vi "读取临时表格数据 (子VI).vi"(8 "time 2":string, 9 "表格选择":string(combo)="database1.mdb", 10 "组合框":string(combo), 11 "String输入":refnum<vi>) -> ()   [LabVIEW 2016]
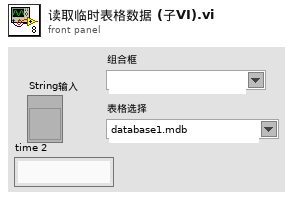
[diagram p1: front panel]
types:
  T1 = enum16{"CODMn", "PH", "氨氮", "总氮", "总磷", "CODCr", "电导率", "水温", "DO", "浊度", "叶绿素", "藻密度"}
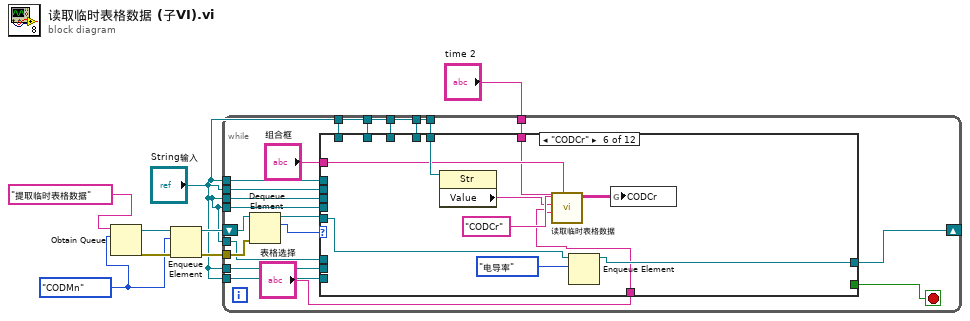
[diagram p0: block diagram]
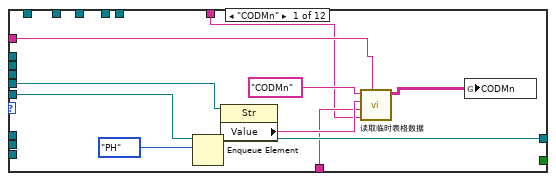
[diagram p2: hidden frame]
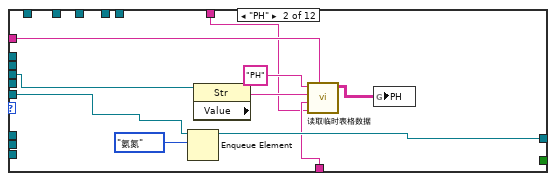
[diagram p3: hidden frame]
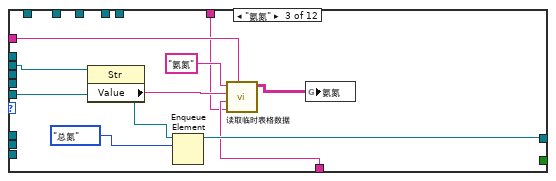
[diagram p4: hidden frame]
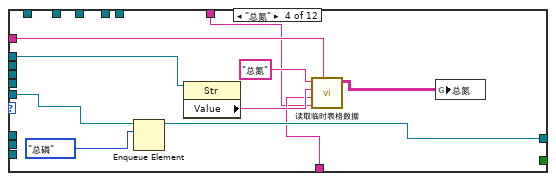
[diagram p5: hidden frame]
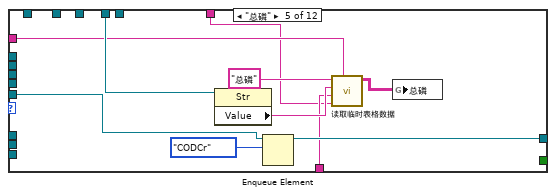
[diagram p6: hidden frame]
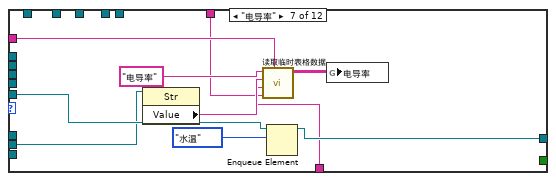
[diagram p7: hidden frame]
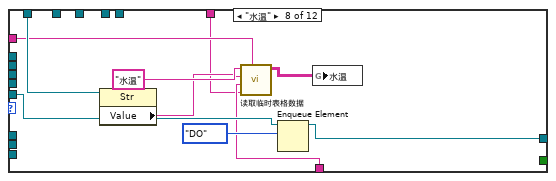
[diagram p8: hidden frame]
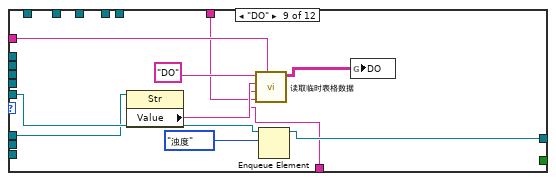
[diagram p9: hidden frame]
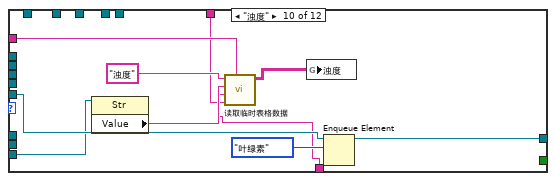
[diagram p10: hidden frame]
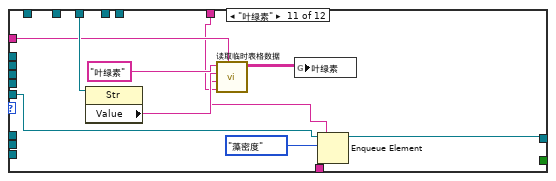
[diagram p11: hidden frame]
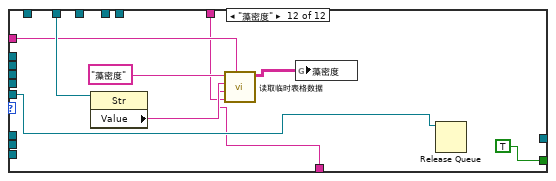
[diagram p12: hidden frame]
diagram:
  w4 = T1."CODMn"
  n1 = Obtain Queue(name (unnamed)="提取临时表格数据" ("新元素/子数组"), element data type=w4) -> (queue out=w8:refnum<queue>, error out=w5:errorcluster)  [unwired: 3 in, 1 out]
  n2 = Enqueue Element(queue=w8, element=w4, error in (no error)=w5) -> (queue out=w7:refnum<queue>, error out=w6:errorcluster)  [unwired: 1 in, 1 out]
  n3 = while {
    shift-right: [w27] -> _
    shift-left: w7 -> [w29]
    tunnel: w6 -> [w26]
    tunnel: "String输入" -> [w23]
    tunnel: "String输入" -> [w22]
    tunnel: "String输入" -> [w21]
    tunnel: "String输入" -> [w20]
    tunnel: "String输入" -> [w19]
    tunnel: "String输入" -> [w18]
    tunnel: "String输入" -> [w17]
    tunnel: "String输入" -> [w16]
    tunnel: "String输入" -> [w15]
    tunnel: "String输入" -> [w14]
    tunnel: "String输入" -> [w13]
    tunnel: "String输入" -> [w12]
    tunnel: "time 2" -> [w9]
    stop <- w24 stop-if-true
    n4 = Dequeue Element(queue=w29, error in (no error)=w26) -> (queue out=w28:refnum<queue>, element=w25:T1)  [unwired: 1 in, 2 out]
    n5 = case shown="\"CODCr\"" w25 {
      tunnel: w28 -> [w39 w49 w58 w69 w78 w88 w98 w108 w118 w128 w138 w147]
      tunnel: [w38 w48 w59 w68 w77 w87 w97 w107 w117 w127 w137 _] -> w27
      tunnel: [_ _ _ _ _ _ _ _ _ _ _ TRUE] -> w24
      tunnel: w23 -> [w33 _ _ _ _ _ _ _ _ _ _ _]
      tunnel: w22 -> [_ w43 _ _ _ _ _ _ _ _ _ _]
      tunnel: w21 -> [_ _ w53 _ _ _ _ _ _ _ _ _]
      tunnel: w20 -> [_ _ _ w63 _ _ _ _ _ _ _ _]
      tunnel: w19 -> [_ _ _ _ w73 _ _ _ _ _ _ _]
      tunnel: w18 -> [_ _ _ _ _ w83 _ _ _ _ _ _]
      tunnel: w17 -> [_ _ _ _ _ _ w93 _ _ _ _ _]
      tunnel: w16 -> [_ _ _ _ _ _ _ w103 _ _ _ _]
      tunnel: w15 -> [_ _ _ _ _ _ _ _ w113 _ _ _]
      tunnel: w14 -> [_ _ _ _ _ _ _ _ _ w123 _ _]
      tunnel: w13 -> [_ _ _ _ _ _ _ _ _ _ w133 _]
      tunnel: w12 -> [_ _ _ _ _ _ _ _ _ _ _ w143]
      tunnel: "组合框" -> [w32 w42 w52 w62 w72 w82 w92 w102 w112 w122 w132 w142]
      tunnel: "表格选择" -> [w31 w41 w51 w61 w71 w81 w91 w101 w111 w121 w131 w141]
      tunnel: w9 -> [w30 w40 w50 w60 w70 w80 w90 w100 w110 w120 w130 w140]
      frame "CODMn" {
        n6 = Enqueue Element(queue=w39, element=T1."PH") -> (queue out=w38:refnum<queue>)  [unwired: 2 in, 2 out]
        n7 = property class="Str"(reference=w33) -> ("Value"=w35:string)  [unwired: 1 in, 2 out]
        n8 = call "读取临时表格数据.vi"("组合框"=w32, "time 2"=w30, "表格选择"=w31, "time"=w35, "table输入"="CODMn" ("元素")) -> ("data"=w34:string[][])  [unwired: 5 in, 1 out]
        n9 = global write "全局 所有参数.vi" "CODMn"(w34) -> ()
      }
      frame "PH" {
        n10 = Enqueue Element(queue=w49, element=T1."氨氮") -> (queue out=w48:refnum<queue>)  [unwired: 2 in, 2 out]
        n11 = property class="Str"(reference=w43) -> ("Value"=w45:string)  [unwired: 1 in, 2 out]
        n12 = call "读取临时表格数据.vi"("组合框"=w42, "time 2"=w40, "表格选择"=w41, "time"=w45, "table输入"="PH" ("元素")) -> ("data"=w44:string[][])  [unwired: 5 in, 1 out]
        n13 = global write "全局 所有参数.vi" "PH"(w44) -> ()
      }
      frame "氨氮" {
        n14 = property class="Str"(reference=w53) -> ("Value"=w55:string)  [unwired: 1 in, 2 out]
        n15 = Enqueue Element(queue=w58, element=T1."总氮") -> (queue out=w59:refnum<queue>)  [unwired: 2 in, 2 out]
        n16 = call "读取临时表格数据.vi"("组合框"=w52, "time 2"=w50, "表格选择"=w51, "time"=w55, "table输入"="氨氮" ("元素")) -> ("data"=w54:string[][])  [unwired: 5 in, 1 out]
        n17 = global write "全局 所有参数.vi" "氨氮"(w54) -> ()
      }
      frame "总氮" {
        n18 = Enqueue Element(queue=w69, element=T1."总磷") -> (queue out=w68:refnum<queue>)  [unwired: 2 in, 2 out]
        n19 = property class="Str"(reference=w63) -> ("Value"=w65:string)  [unwired: 1 in, 2 out]
        n20 = call "读取临时表格数据.vi"("组合框"=w62, "time 2"=w60, "表格选择"=w61, "time"=w65, "table输入"="总氮" ("元素")) -> ("data"=w64:string[][])  [unwired: 5 in, 1 out]
        n21 = global write "全局 所有参数.vi" "总氮"(w64) -> ()
      }
      frame "总磷" {
        n22 = property class="Str"(reference=w73) -> ("Value"=w75:string)  [unwired: 1 in, 2 out]
        n23 = Enqueue Element(queue=w78, element=T1."CODCr") -> (queue out=w77:refnum<queue>)  [unwired: 2 in, 2 out]
        n24 = call "读取临时表格数据.vi"("组合框"=w72, "time 2"=w70, "表格选择"=w71, "time"=w75, "table输入"="总磷" ("元素")) -> ("data"=w74:string[][])  [unwired: 5 in, 1 out]
        n25 = global write "全局 所有参数.vi" "总磷"(w74) -> ()
      }
      frame "CODCr" {
        n26 = property class="Str"(reference=w83) -> ("Value"=w85:string)  [unwired: 1 in, 2 out]
        n27 = call "读取临时表格数据.vi"("组合框"=w82, "time 2"=w80, "表格选择"=w81, "time"=w85, "table输入"="CODCr" ("元素")) -> ("data"=w84:string[][])  [unwired: 5 in, 1 out]
        n28 = Enqueue Element(queue=w88, element=T1."电导率") -> (queue out=w87:refnum<queue>)  [unwired: 2 in, 2 out]
        n29 = global write "全局 所有参数.vi" "CODCr"(w84) -> ()
      }
      frame "电导率" {
        n30 = property class="Str"(reference=w93) -> ("Value"=w95:string)  [unwired: 1 in, 2 out]
        n31 = call "读取临时表格数据.vi"("组合框"=w92, "time 2"=w90, "表格选择"=w91, "time"=w95, "table输入"="电导率" ("元素")) -> ("data"=w94:string[][])  [unwired: 5 in, 1 out]
        n32 = Enqueue Element(queue=w98, element=T1."水温") -> (queue out=w97:refnum<queue>)  [unwired: 2 in, 2 out]
        n33 = global write "全局 所有参数.vi" "电导率"(w94) -> ()
      }
      frame "水温" {
        n34 = property class="Str"(reference=w103) -> ("Value"=w105:string)  [unwired: 1 in, 2 out]
        n35 = call "读取临时表格数据.vi"("组合框"=w102, "time 2"=w100, "表格选择"=w101, "time"=w105, "table输入"="水温" ("元素")) -> ("data"=w104:string[][])  [unwired: 5 in, 1 out]
        n36 = Enqueue Element(queue=w108, element=T1."DO") -> (queue out=w107:refnum<queue>)  [unwired: 2 in, 2 out]
        n37 = global write "全局 所有参数.vi" "水温"(w104) -> ()
      }
      frame "DO" {
        n38 = property class="Str"(reference=w113) -> ("Value"=w115:string)  [unwired: 1 in, 2 out]
        n39 = call "读取临时表格数据.vi"("组合框"=w112, "time 2"=w110, "表格选择"=w111, "time"=w115, "table输入"="DO" ("元素")) -> ("data"=w114:string[][])  [unwired: 5 in, 1 out]
        n40 = Enqueue Element(queue=w118, element=T1."浊度") -> (queue out=w117:refnum<queue>)  [unwired: 2 in, 2 out]
        n41 = global write "全局 所有参数.vi" "DO"(w114) -> ()
      }
      frame "浊度" {
        n42 = property class="Str"(reference=w123) -> ("Value"=w124:string)  [unwired: 1 in, 2 out]
        n43 = call "读取临时表格数据.vi"("组合框"=w122, "time 2"=w120, "表格选择"=w121, "time"=w124, "table输入"="浊度" ("元素")) -> ("data"=w126:string[][])  [unwired: 5 in, 1 out]
        n44 = global write "全局 所有参数.vi" "浊度"(w126) -> ()
        n45 = Enqueue Element(queue=w128, element=T1."叶绿素") -> (queue out=w127:refnum<queue>)  [unwired: 2 in, 2 out]
      }
      frame "叶绿素" {
        n46 = property class="Str"(reference=w133) -> ("Value"=w135:string)  [unwired: 1 in, 2 out]
        n47 = call "读取临时表格数据.vi"("组合框"=w132, "time 2"=w130, "表格选择"=w131, "time"=w135, "table输入"="叶绿素" ("元素")) -> ("data"=w134:string[][])  [unwired: 5 in, 1 out]
        n48 = global write "全局 所有参数.vi" "叶绿素"(w134) -> ()
        n49 = Enqueue Element(queue=w138, element=T1."藻密度") -> (queue out=w137:refnum<queue>)  [unwired: 2 in, 2 out]
      }
      frame "藻密度" {
        n50 = property class="Str"(reference=w143) -> ("Value"=w145:string)  [unwired: 1 in, 2 out]
        n51 = call "读取临时表格数据.vi"("组合框"=w142, "time 2"=w140, "表格选择"=w141, "time"=w145, "table输入"="藻密度" ("元素")) -> ("data"=w144:string[][])  [unwired: 5 in, 1 out]
        n52 = global write "全局 所有参数.vi" "藻密度"(w144) -> ()
        n53 = Release Queue(queue=w147) -> ()  [unwired: 2 in, 3 out]
      }
    }
  }
